vi "Write Live Preview Timeout.vi"(8 "error in (no error)":errorcluster, 10 "Live Preview Timeout":i32, 11 "Virtual Camera in":refnum<class "Virtual Camera.lvclass">) -> (0 "error out":errorcluster, 3 "Virtual Camera out":refnum<class "Virtual Camera.lvclass">)   [LabVIEW 2018]
uses:
  Virtual Camera.lvclass
  C:/LVCUR/flash-gordon/Hardware/Camera/Camera.lvclass
  C:/LVCUR/flash-gordon/Hardware/Device/Device.lvclass
  C:/Program Files/National Instruments/LabVIEW 2018/vi.lib/ActorFramework/Actor/Actor.lvclass
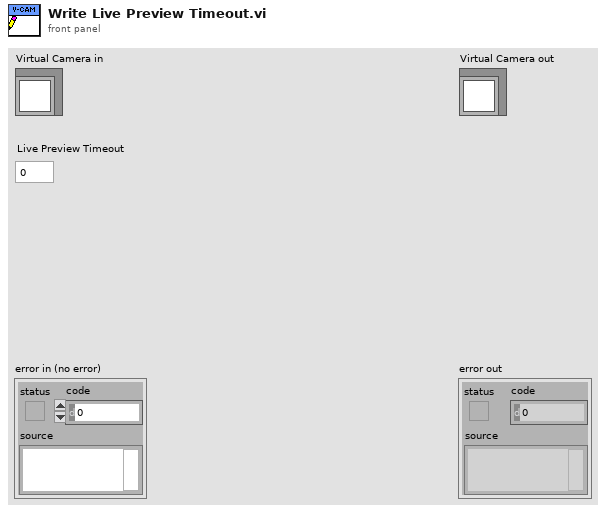
[diagram p1: front panel]
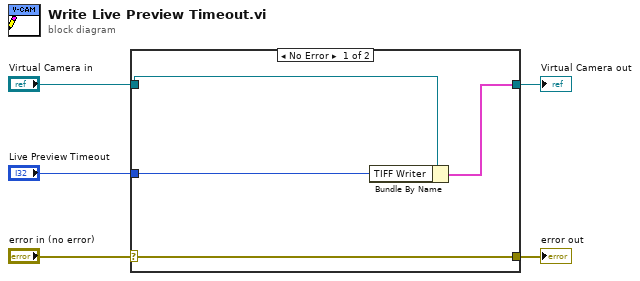
[diagram p0: block diagram]
diagram:
  n1 = case shown="No Error" "error in (no error)" {
    selector: "error in (no error)" -> [w9 w10]
    tunnel: [w9 w10] -> w4
    tunnel: [w7 w11] -> w2
    tunnel: "Virtual Camera in" -> [w8 w11]
    tunnel: "Live Preview Timeout" -> [w6 _]
    frame No Error {
      n2 = Bundle By Name(cluster=w8, "TIFF Writer"=w6) -> (w7:cluster{})
    }
    frame Error {
    }
  }
  "error out" <- w4
  "Virtual Camera out" <- w2
